vi "Unit conversion.vi"() -> ()   [LabVIEW 2016]
uses:
  <vilib>/express/express arith-compare/Formula/XNode/ExpressFormulaBlockNode.xnode
panel:
  out "converted":dbl
  in  "Ring":u16(ring) items=["lbm", "slugs"]
  in  "Mass (kg)":dbl
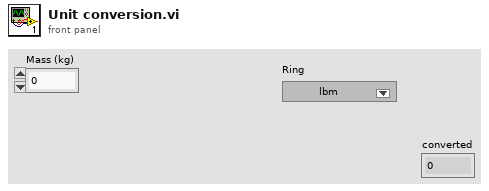
[diagram p1: front panel]
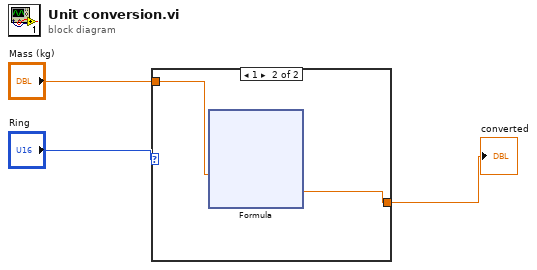
[diagram p0: block diagram]
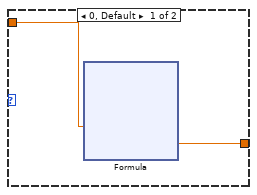
[diagram p2: hidden frame]
diagram:
  n1 = case shown="1" "Ring" {
    tunnel: [w4 w14] -> w2
    tunnel: "Mass (kg)" -> [w5 w15]
    frame 0, Default {
      n2 = xnode "Formula"("kg"=w5) -> ("Result"=w4:dbl)  [unwired: 1 in, 1 out]
    }
    frame 1 {
      n3 = xnode "Formula"("kg"=w15) -> ("Result"=w14:dbl)  [unwired: 1 in, 1 out]
    }
  }
  "converted" <- w2
